vi "Read Sender.vi"(11 "Terminated Msg in":refnum<class "Terminated Msg.lvclass">) -> (2 "Sender":refnum<class "Sender.lvclass">)   [LabVIEW 2025, in "jettl.lvlib" / "Terminated Msg.lvlib" / "Terminated Msg.lvclass"]
uses:
  Terminated Msg.lvclass
  Terminated Msg.lvclass/Terminated Msg.ctl
  Sender/Sender/Sender.lvclass
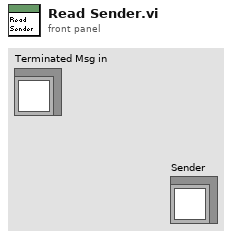
[diagram p1: front panel]
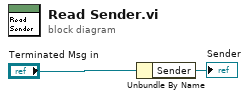
[diagram p0: block diagram]
diagram:
  n1 = Unbundle By Name("Terminated Msg in") -> ("Sender"=→"Sender":refnum<class "Sender.lvclass">)
